vi "input_channel_to_json.vi"(1 "Analog Input Channels":T1[](array[typedef])=[{"Input Type"=enum."DAQ", "Channel Name"="Vapor Mass Flow", "Physical Channel"="cDAQ1Mod2/ai5", "Sensor Type"=enum."Mass Flow Rate", "Signal Type"=enum."Current", "Terminal Configuration"=-1, "Minimum Value"=0.004, "Maximum Value"=0.02, "TC Type"=10086, "Sensor Min"=0.0, "Sensor Max"=377.9933, "Sensor Offset"=0.0, "Sensor Unit"=enum."g/s", "Output Unit"=enum."g/s", "Unit Conversion"=1.0, "Active"=TRUE}, {"Input Type"=enum."DAQ", "Channel Name"="Vapor Line Density", "Physical Channel"="cDAQ1Mod2/ai6", "Sensor Type"=enum."Density", "Signal Type"=enum."Current", "Terminal Configuration"=-1, "Minimum Value"=0.004, "Maximum Value"=0.02, "TC Type"=10086, "Sensor Min"=0.0, "Sensor Max"=2.0, "Sensor Offset"=0.0, "Sensor Unit"=enum."g/cm3", "Output Unit"=enum."g/cm3", "Unit Conversion"=1.0, "Active"=TRUE}, {"Input Type"=enum."DAQ", "Channel Name"="Liquid Mass Flow", "Physical Channel"="cDAQ1Mod2/ai3", "Sensor Type"=enum."Mass Flow Rate", "Signal Type"=enum."Current", "Terminal Configuration"=-1, "Minimum Value"=0.004, "Maximum Value"=0.02, "TC Type"=10086, "Sensor Min"=0.0, "Sensor Max"=377.9933, "Sensor Offset"=0.0, "Sensor Unit"=enum."g/s", "Output Unit"=enum."g/s", "Unit Conversion"=1.0, "Active"=TRUE}, {"Input Type"=enum."DAQ", "Channel Name"="Liquid Line Density", "Physical Channel"="cDAQ1Mod2/ai4", "Sensor Type"=enum."Density", "Signal Type"=enum."Current", "Terminal Configuration"=-1, "Minimum Value"=0.004, "Maximum Value"=0.02, "TC Type"=10086, "Sensor Min"=0.0, "Sensor Max"=2.0, "Sensor Offset"=0.0, "Sensor Unit"=enum."g/cm3", "Output Unit"=enum."g/cm3", "Unit Conversion"=1.0, "Active"=TRUE}, {"Input Type"=enum."DAQ", "Channel Name"="Vapor Inlet Pressure DEPR", "Physical Channel"="cDAQ1Mod5/ai1", "Sensor Type"=enum."Absolute Pressure", "Signal Type"=enum."Voltage", "Terminal Configuration"=10078, "Minimum Value"=0.0, "Maximum Value"=5.0, "TC Type"=10086, "Sensor Min"=0.0, "Sensor Max"=50.0, "Sensor Offset"=0.0, "Sensor Unit"=enum."psi", "Output Unit"=enum."Pa", "Unit Conversion"=6894.75729, "Active"=FALSE}, {"Input Type"=enum."DAQ", "Channel Name"="Mega Tank Pressure", "Physical Channel"="cDAQ1Mod5/ai2", "Sensor Type"=enum."Absolute Pressure", "Signal Type"=enum."Voltage", "Terminal Configuration"=10078, "Minimum Value"=0.5, "Maximum Value"=5.5, "TC Type"=10086, "Sensor Min"=0.0, "Sensor Max"=50.0, "Sensor Offset"=0.0, "Sensor Unit"=enum."psi", "Output Unit"=enum."Pa", "Unit Conversion"=6894.75729, "Active"=TRUE}, {"Input Type"=enum."DAQ", "Channel Name"="Separator Pressure", "Physical Channel"="cDAQ1Mod5/ai0", "Sensor Type"=enum."Absolute Pressure", "Signal Type"=enum."Voltage", "Terminal Configuration"=10078, "Minimum Value"=0.0, "Maximum Value"=5.0, "TC Type"=10086, "Sensor Min"=0.0, "Sensor Max"=50.0, "Sensor Offset"=0.0, "Sensor Unit"=enum."psi", "Output Unit"=enum."Pa", "Unit Conversion"=6894.75729, "Active"=TRUE}, {"Input Type"=enum."DAQ", "Channel Name"="Liquid Inlet Pressure", "Physical Channel"="cDAQ1Mod5/ai4", "Sensor Type"=enum."Absolute Pressure", "Signal Type"=enum."Voltage", "Terminal Configuration"=10078, "Minimum Value"=0.0, "Maximum Value"=5.0, "TC Type"=10086, "Sensor Min"=0.0, "Sensor Max"=50.0, "Sensor Offset"=0.0, "Sensor Unit"=enum."psi", "Output Unit"=enum."Pa", "Unit Conversion"=6894.75729, "Active"=TRUE}, {"Input Type"=enum."DAQ", "Channel Name"="Vapor Inlet Pressure ", "Physical Channel"="cDAQ1Mod5/ai3", "Sensor Type"=enum."Absolute Pressure", "Signal Type"=enum."Voltage", "Terminal Configuration"=10078, "Minimum Value"=0.0, "Maximum Value"=5.0, "TC Type"=10086, "Sensor Min"=0.0, "Sensor Max"=50.0, "Sensor Offset"=0.0, "Sensor Unit"=enum."psi", "Output Unit"=enum."Pa", "Unit Conversion"=6894.75729, "Active"=TRUE}, {"Input Type"=enum."DAQ", "Channel Name"="Vapor Inlet Temperature", "Physical Channel"="cDAQ1Mod6/ai1", "Sensor Type"=enum."Temperature", "Signal Type"=enum."Temperature", "Terminal Configuration"=-1, "Minimum Value"=0.0, "Maximum Value"=100.0, "TC Type"=10086, "Sensor Min"=0.0, "Sensor Max"=100.0, "Sensor Offset"=0.0, "Sensor Unit"=enum."C", "Output Unit"=enum."C", "Unit Conversion"=1.0, "Active"=TRUE}, {"Input Type"=enum."DAQ", "Channel Name"="Vapor Inlet Temperature DEPR", "Physical Channel"="cDAQ1Mod7/ai0", "Sensor Type"=enum."Temperature", "Signal Type"=enum."Temperature", "Terminal Configuration"=-1, "Minimum Value"=0.0, "Maximum Value"=100.0, "TC Type"=10086, "Sensor Min"=0.0, "Sensor Max"=100.0, "Sensor Offset"=0.0, "Sensor Unit"=enum."C", "Output Unit"=enum."C", "Unit Conversion"=1.0, "Active"=FALSE}, {"Input Type"=enum."DAQ", "Channel Name"="Mega Tank Temperature", "Physical Channel"="cDAQ1Mod6/ai2", "Sensor Type"=enum."Temperature", "Signal Type"=enum."Temperature", "Terminal Configuration"=-1, "Minimum Value"=0.0, "Maximum Value"=100.0, "TC Type"=10086, "Sensor Min"=0.0, "Sensor Max"=100.0, "Sensor Offset"=0.0, "Sensor Unit"=enum."C", "Output Unit"=enum."C", "Unit Conversion"=1.0, "Active"=TRUE}, {"Input Type"=enum."DAQ", "Channel Name"="Liquid Inlet Temperature", "Physical Channel"="cDAQ1Mod7/ai3", "Sensor Type"=enum."Temperature", "Signal Type"=enum."Temperature", "Terminal Configuration"=-1, "Minimum Value"=0.0, "Maximum Value"=100.0, "TC Type"=10086, "Sensor Min"=0.0, "Sensor Max"=100.0, "Sensor Offset"=0.0, "Sensor Unit"=enum."C", "Output Unit"=enum."C", "Unit Conversion"=1.0, "Active"=TRUE}, {"Input Type"=enum."DAQ", "Channel Name"="Separator Temperature", "Physical Channel"="cDAQ1Mod6/ai0", "Sensor Type"=enum."Temperature", "Signal Type"=enum."Temperature", "Terminal Configuration"=-1, "Minimum Value"=0.0, "Maximum Value"=100.0, "TC Type"=10086, "Sensor Min"=0.0, "Sensor Max"=100.0, "Sensor Offset"=0.0, "Sensor Unit"=enum."C", "Output Unit"=enum."C", "Unit Conversion"=1.0, "Active"=TRUE}, {"Input Type"=enum."DAQ", "Channel Name"="Lower Dev Section Pressure", "Physical Channel"="cDAQ1Mod5/ai6", "Sensor Type"=enum."Absolute Pressure", "Signal Type"=enum."Voltage", "Terminal Configuration"=10078, "Minimum Value"=0.0, "Maximum Value"=5.0, "TC Type"=10086, "Sensor Min"=0.0, "Sensor Max"=60.0, "Sensor Offset"=0.0, "Sensor Unit"=enum."psi", "Output Unit"=enum."Pa", "Unit Conversion"=6894.75729, "Active"=TRUE}, {"Input Type"=enum."DAQ", "Channel Name"="Upper Dev Section Temperature", "Physical Channel"="cDAQ1Mod6/ai3", "Sensor Type"=enum."Temperature", "Signal Type"=enum."Temperature", "Terminal Configuration"=-1, "Minimum Value"=0.0, "Maximum Value"=100.0, "TC Type"=10086, "Sensor Min"=0.0, "Sensor Max"=100.0, "Sensor Offset"=0.0, "Sensor Unit"=enum."C", "Output Unit"=enum."C", "Unit Conversion"=1.0, "Active"=TRUE}, {"Input Type"=enum."DAQ", "Channel Name"="Upper Dev Section Pressure", "Physical Channel"="cDAQ1Mod5/ai5", "Sensor Type"=enum."Absolute Pressure", "Signal Type"=enum."Voltage", "Terminal Configuration"=10078, "Minimum Value"=0.0, "Maximum Value"=5.0, "TC Type"=10086, "Sensor Min"=0.0, "Sensor Max"=60.0, "Sensor Offset"=0.0, "Sensor Unit"=enum."psi", "Output Unit"=enum."Pa", "Unit Conversion"=6894.75729, "Active"=TRUE}, {"Input Type"=enum."DAQ", "Channel Name"="Test Section Temperature", "Physical Channel"="cDAQ1Mod6/ai10", "Sensor Type"=enum."Temperature", "Signal Type"=enum."Temperature", "Terminal Configuration"=-1, "Minimum Value"=0.0, "Maximum Value"=100.0, "TC Type"=10086, "Sensor Min"=0.0, "Sensor Max"=100.0, "Sensor Offset"=0.0, "Sensor Unit"=enum."C", "Output Unit"=enum."C", "Unit Conversion"=1.0, "Active"=TRUE}, {"Input Type"=enum."DAQ", "Channel Name"="Test Section Pressure", "Physical Channel"="cDAQ1Mod5/ai7", "Sensor Type"=enum."Absolute Pressure", "Signal Type"=enum."Voltage", "Terminal Configuration"=10078, "Minimum Value"=0.0, "Maximum Value"=5.0, "TC Type"=10086, "Sensor Min"=0.0, "Sensor Max"=50.0, "Sensor Offset"=0.0, "Sensor Unit"=enum."psi", "Output Unit"=enum."Pa", "Unit Conversion"=6894.75729, "Active"=TRUE}, {"Input Type"=enum."DAQ", "Channel Name"="Dwyer dP DEPR", "Physical Channel"="cDAQ1Mod5/ai9", "Sensor Type"=enum."Differential Pressure", "Signal Type"=enum."Voltage", "Terminal Configuration"=10078, "Minimum Value"=0.05, "Maximum Value"=5.05, "TC Type"=10086, "Sensor Min"=0.0, "Sensor Max"=1.0, "Sensor Offset"=0.0, "Sensor Unit"=enum."psi", "Output Unit"=enum."Pa", "Unit Conversion"=6894.75729, "Active"=FALSE}, {"Input Type"=enum."DAQ", "Channel Name"="Venturi dP", "Physical Channel"="cDAQ1Mod9/ai0", "Sensor Type"=enum."Differential Pressure", "Signal Type"=enum."Current", "Terminal Configuration"=10083, "Minimum Value"=0.00403, "Maximum Value"=0.02, "TC Type"=10086, "Sensor Min"=0.0, "Sensor Max"=10.0, "Sensor Offset"=0.0, "Sensor Unit"=enum."inH2O", "Output Unit"=enum."Pa", "Unit Conversion"=248.84, "Active"=TRUE}, {"Input Type"=enum."DAQ", "Channel Name"="PGminiPressure", "Physical Channel"="cDAQ1Mod5/ai10", "Sensor Type"=enum."Absolute Pressure", "Signal Type"=enum."Voltage", "Terminal Configuration"=10078, "Minimum Value"=0.0, "Maximum Value"=5.0, "TC Type"=10086, "Sensor Min"=0.0, "Sensor Max"=50.0, "Sensor Offset"=0.0, "Sensor Unit"=enum."psi", "Output Unit"=enum."Pa", "Unit Conversion"=6894.75729, "Active"=TRUE}, {"Input Type"=enum."DAQ", "Channel Name"="PGminiTemperature", "Physical Channel"="cDAQ1Mod7/ai6", "Sensor Type"=enum."Temperature", "Signal Type"=enum."Temperature", "Terminal Configuration"=-1, "Minimum Value"=0.0, "Maximum Value"=100.0, "TC Type"=10073, "Sensor Min"=0.0, "Sensor Max"=100.0, "Sensor Offset"=0.0, "Sensor Unit"=enum."C", "Output Unit"=enum."C", "Unit Conversion"=1.0, "Active"=TRUE}, {"Input Type"=enum."DAQ", "Channel Name"="Atmospheric Pressure", "Physical Channel"="cDAQ1Mod5/ai8", "Sensor Type"=enum."Absolute Pressure", "Signal Type"=enum."Voltage", "Terminal Configuration"=10078, "Minimum Value"=1.0, "Maximum Value"=5.0, "TC Type"=10086, "Sensor Min"=0.0, "Sensor Max"=25.0, "Sensor Offset"=0.0, "Sensor Unit"=enum."psi", "Output Unit"=enum."Pa", "Unit Conversion"=6894.75729, "Active"=TRUE}, {"Input Type"=enum."DAQ", "Channel Name"="PG Absolute Pressure", "Physical Channel"="cDAQ1Mod5/ai11", "Sensor Type"=enum."Absolute Pressure", "Signal Type"=enum."Voltage", "Terminal Configuration"=10078, "Minimum Value"=0.0, "Maximum Value"=5.0, "TC Type"=10086, "Sensor Min"=0.0, "Sensor Max"=60.0, "Sensor Offset"=0.0, "Sensor Unit"=enum."psi", "Output Unit"=enum."Pa", "Unit Conversion"=6894.75729, "Active"=TRUE}, {"Input Type"=enum."DAQ", "Channel Name"="Dwyer dP", "Physical Channel"="cDAQ1Mod2/ai7", "Sensor Type"=enum."Differential Pressure", "Signal Type"=enum."Current", "Terminal Configuration"=-1, "Minimum Value"=0.004, "Maximum Value"=0.02, "TC Type"=10086, "Sensor Min"=0.0, "Sensor Max"=500.0, "Sensor Offset"=0.0, "Sensor Unit"=enum."Pa", "Output Unit"=enum."Pa", "Unit Conversion"=1.0, "Active"=TRUE}, {"Input Type"=enum."DAQ", "Channel Name"="Mixing Tee dP DEPR", "Physical Channel"="", "Sensor Type"=enum."Differential Pressure", "Signal Type"=enum."Current", "Terminal Configuration"=-1, "Minimum Value"=0.004, "Maximum Value"=0.02, "TC Type"=10086, "Sensor Min"=0.0, "Sensor Max"=50.0, "Sensor Offset"=0.0, "Sensor Unit"=enum."psi", "Output Unit"=enum."Pa", "Unit Conversion"=6894.75729, "Active"=FALSE}, {"Input Type"=enum."DAQ", "Channel Name"="PG Vapor Temperature", "Physical Channel"="cDAQ1Mod7/ai4", "Sensor Type"=enum."Temperature", "Signal Type"=enum."Temperature", "Terminal Configuration"=-1, "Minimum Value"=0.0, "Maximum Value"=100.0, "TC Type"=10073, "Sensor Min"=0.0, "Sensor Max"=100.0, "Sensor Offset"=0.0, "Sensor Unit"=enum."C", "Output Unit"=enum."C", "Unit Conversion"=1.0, "Active"=TRUE}, {"Input Type"=enum."DAQ", "Channel Name"="PG Liquid Temperature", "Physical Channel"="cDAQ1Mod7/ai5", "Sensor Type"=enum."Temperature", "Signal Type"=enum."Temperature", "Terminal Configuration"=-1, "Minimum Value"=0.0, "Maximum Value"=100.0, "TC Type"=10073, "Sensor Min"=0.0, "Sensor Max"=100.0, "Sensor Offset"=0.0, "Sensor Unit"=enum."C", "Output Unit"=enum."C", "Unit Conversion"=1.0, "Active"=TRUE}, {"Input Type"=enum."DAQ", "Channel Name"="Window 1 to 4 dP", "Physical Channel"="cDAQ1Mod2/ai2", "Sensor Type"=enum."Differential Pressure", "Signal Type"=enum."Current", "Terminal Configuration"=-1, "Minimum Value"=0.004, "Maximum Value"=0.02, "TC Type"=10086, "Sensor Min"=0.0, "Sensor Max"=20.0, "Sensor Offset"=0.0, "Sensor Unit"=enum."inH2O", "Output Unit"=enum."Pa", "Unit Conversion"=248.84, "Active"=TRUE}, {"Input Type"=enum."DAQ", "Channel Name"="Window 1 to 7 dP", "Physical Channel"="cDAQ1Mod2/ai1", "Sensor Type"=enum."Differential Pressure", "Signal Type"=enum."Current", "Terminal Configuration"=-1, "Minimum Value"=0.004, "Maximum Value"=0.02, "TC Type"=10086, "Sensor Min"=0.0, "Sensor Max"=20.0, "Sensor Offset"=0.0, "Sensor Unit"=enum."inH2O", "Output Unit"=enum."Pa", "Unit Conversion"=248.84, "Active"=TRUE}, {"Input Type"=enum."DAQ", "Channel Name"="Window 1 to 7 Fast dP", "Physical Channel"="cDAQ1Mod2/ai0", "Sensor Type"=enum."Differential Pressure", "Signal Type"=enum."Current", "Terminal Configuration"=-1, "Minimum Value"=0.004, "Maximum Value"=0.02, "TC Type"=10086, "Sensor Min"=0.0, "Sensor Max"=2.5, "Sensor Offset"=0.0, "Sensor Unit"=enum."psi", "Output Unit"=enum."Pa", "Unit Conversion"=6894.75729, "Active"=TRUE}, {"Input Type"=enum."DAQ", "Channel Name"="Camera Voltage", "Physical Channel"="cDAQ1Mod8/ai0", "Sensor Type"=enum."Other", "Signal Type"=enum."Voltage", "Terminal Configuration"=10106, "Minimum Value"=0.0, "Maximum Value"=10.0, "TC Type"=10086, "Sensor Min"=0.0, "Sensor Max"=50.0, "Sensor Offset"=0.0, "Sensor Unit"=enum."Volt", "Output Unit"=enum."Volt", "Unit Conversion"=1.0, "Active"=TRUE}, {"Input Type"=enum."DAQ", "Channel Name"="Tinlet", "Physical Channel"="cDAQ1Mod6/ai4", "Sensor Type"=enum."Temperature", "Signal Type"=enum."Temperature", "Terminal Configuration"=-1, "Minimum Value"=0.0, "Maximum Value"=100.0, "TC Type"=10055, "Sensor Min"=-0.432, "Sensor Max"=99.438, "Sensor Offset"=0.0, "Sensor Unit"=enum."C", "Output Unit"=enum."C", "Unit Conversion"=1.0, "Active"=TRUE}, {"Input Type"=enum."DAQ", "Channel Name"="Tsectwo", "Physical Channel"="cDAQ1Mod6/ai5", "Sensor Type"=enum."Temperature", "Signal Type"=enum."Temperature", "Terminal Configuration"=-1, "Minimum Value"=0.0, "Maximum Value"=100.0, "TC Type"=10055, "Sensor Min"=-0.3803, "Sensor Max"=99.4597, "Sensor Offset"=0.0, "Sensor Unit"=enum."C", "Output Unit"=enum."C", "Unit Conversion"=1.0, "Active"=TRUE}, {"Input Type"=enum."DAQ", "Channel Name"="TS Window 1 Absolute Pressure", "Physical Channel"="cDAQ1Mod5/ai12", "Sensor Type"=enum."Absolute Pressure", "Signal Type"=enum."Voltage", "Terminal Configuration"=10078, "Minimum Value"=0.0, "Maximum Value"=5.0, "TC Type"=10086, "Sensor Min"=0.0, "Sensor Max"=50.0, "Sensor Offset"=0.0, "Sensor Unit"=enum."psi", "Output Unit"=enum."Pa", "Unit Conversion"=6894.75729, "Active"=TRUE}, {"Input Type"=enum."DAQ", "Channel Name"="TS Window 7 Absolute Pressure", "Physical Channel"="cDAQ1Mod5/ai13", "Sensor Type"=enum."Absolute Pressure", "Signal Type"=enum."Voltage", "Terminal Configuration"=10078, "Minimum Value"=0.0, "Maximum Value"=5.0, "TC Type"=10086, "Sensor Min"=0.0, "Sensor Max"=50.0, "Sensor Offset"=0.0, "Sensor Unit"=enum."psi", "Output Unit"=enum."Pa", "Unit Conversion"=6894.75729, "Active"=TRUE}, {"Input Type"=enum."DAQ", "Channel Name"="Liquid Main Diode", "Physical Channel"="cDAQ1Mod10/ai0", "Sensor Type"=enum."Other", "Signal Type"=enum."Voltage", "Terminal Configuration"=10106, "Minimum Value"=0.0, "Maximum Value"=10.0, "TC Type"=10086, "Sensor Min"=0.0, "Sensor Max"=10.0, "Sensor Offset"=0.0, "Sensor Unit"=enum."Volt", "Output Unit"=enum."Volt", "Unit Conversion"=1.0, "Active"=TRUE}, {"Input Type"=enum."DAQ", "Channel Name"="Liquid Control Diode", "Physical Channel"="cDAQ1Mod10/ai1", "Sensor Type"=enum."Other", "Signal Type"=enum."Voltage", "Terminal Configuration"=10106, "Minimum Value"=0.0, "Maximum Value"=10.0, "TC Type"=10086, "Sensor Min"=0.0, "Sensor Max"=10.0, "Sensor Offset"=0.0, "Sensor Unit"=enum."Volt", "Output Unit"=enum."Volt", "Unit Conversion"=1.0, "Active"=TRUE}, {"Input Type"=enum."DAQ", "Channel Name"="Vapor Main Diode", "Physical Channel"="cDAQ1Mod10/ai2", "Sensor Type"=enum."Other", "Signal Type"=enum."Voltage", "Terminal Configuration"=10106, "Minimum Value"=0.0, "Maximum Value"=10.0, "TC Type"=10086, "Sensor Min"=0.0, "Sensor Max"=10.0, "Sensor Offset"=0.0, "Sensor Unit"=enum."Volt", "Output Unit"=enum."Volt", "Unit Conversion"=1.0, "Active"=TRUE}, {"Input Type"=enum."DAQ", "Channel Name"="Vapor Control Diode", "Physical Channel"="cDAQ1Mod10/ai3", "Sensor Type"=enum."Other", "Signal Type"=enum."Voltage", "Terminal Configuration"=10106, "Minimum Value"=0.0, "Maximum Value"=10.0, "TC Type"=10086, "Sensor Min"=0.0, "Sensor Max"=10.0, "Sensor Offset"=0.0, "Sensor Unit"=enum."Volt", "Output Unit"=enum."Volt", "Unit Conversion"=1.0, "Active"=TRUE}, {"Input Type"=enum."DAQ", "Channel Name"="TS Exterior Temperature", "Physical Channel"="cDAQ1Mod6/ai6", "Sensor Type"=enum."Temperature", "Signal Type"=enum."Temperature", "Terminal Configuration"=-1, "Minimum Value"=0.0, "Maximum Value"=100.0, "TC Type"=10073, "Sensor Min"=-0.2775, "Sensor Max"=100.1225, "Sensor Offset"=0.0, "Sensor Unit"=enum."C", "Output Unit"=enum."C", "Unit Conversion"=1.0, "Active"=TRUE}, {"Input Type"=enum."DAQ", "Channel Name"="PG Supply Temperature", "Physical Channel"="cDAQ1Mod6/ai7", "Sensor Type"=enum."Temperature", "Signal Type"=enum."Temperature", "Terminal Configuration"=-1, "Minimum Value"=0.0, "Maximum Value"=100.0, "TC Type"=10073, "Sensor Min"=0.0, "Sensor Max"=100.0, "Sensor Offset"=0.0, "Sensor Unit"=enum."C", "Output Unit"=enum."C", "Unit Conversion"=1.0, "Active"=TRUE}, {"Input Type"=enum."DAQ", "Channel Name"="Post Mixing Tee Temperature", "Physical Channel"="cDAQ1Mod7/ai2", "Sensor Type"=enum."Temperature", "Signal Type"=enum."Temperature", "Terminal Configuration"=-1, "Minimum Value"=0.0, "Maximum Value"=100.0, "TC Type"=10073, "Sensor Min"=0.0, "Sensor Max"=1000.0, "Sensor Offset"=0.0, "Sensor Unit"=enum."Volt", "Output Unit"=enum."Volt", "Unit Conversion"=1.0, "Active"=TRUE}, {"Input Type"=enum."DAQ", "Channel Name"="Tsecthree", "Physical Channel"="cDAQ1Mod6/ai8", "Sensor Type"=enum."Temperature", "Signal Type"=enum."Temperature", "Terminal Configuration"=-1, "Minimum Value"=0.0, "Maximum Value"=100.0, "TC Type"=10055, "Sensor Min"=-0.2553, "Sensor Max"=99.6347, "Sensor Offset"=0.0, "Sensor Unit"=enum."C", "Output Unit"=enum."C", "Unit Conversion"=1.0, "Active"=TRUE}, {"Input Type"=enum."DAQ", "Channel Name"="Toutlet", "Physical Channel"="cDAQ1Mod6/ai9", "Sensor Type"=enum."Temperature", "Signal Type"=enum."Temperature", "Terminal Configuration"=-1, "Minimum Value"=0.0, "Maximum Value"=100.0, "TC Type"=10055, "Sensor Min"=-0.1957, "Sensor Max"=99.8043, "Sensor Offset"=0.0, "Sensor Unit"=enum."C", "Output Unit"=enum."C", "Unit Conversion"=1.0, "Active"=TRUE}] {"Unit Conversion" format="%0.5f"; "TC Type" items=["J"=10072, "K"=10073, "N"=10077, "R"=10082, "S"=10085, "T"=10086, "B"=10047, "E"=10055]; "Sensor Offset" format="%0.5f"; "Sensor Max" format="%0.5f"; "Sensor Min" format="%0.5f"; "Maximum Value" format="%.6f"; "Minimum Value" format="%.6f"; "Terminal Configuration" items=["Default"=-1, "RSE"=10083, "NRSE"=10078, "Differential"=10106, "Pseudodifferential"=12529]}) -> (0 "JSON string":string)   [LabVIEW 2017]
uses:
  input_channel.ctl
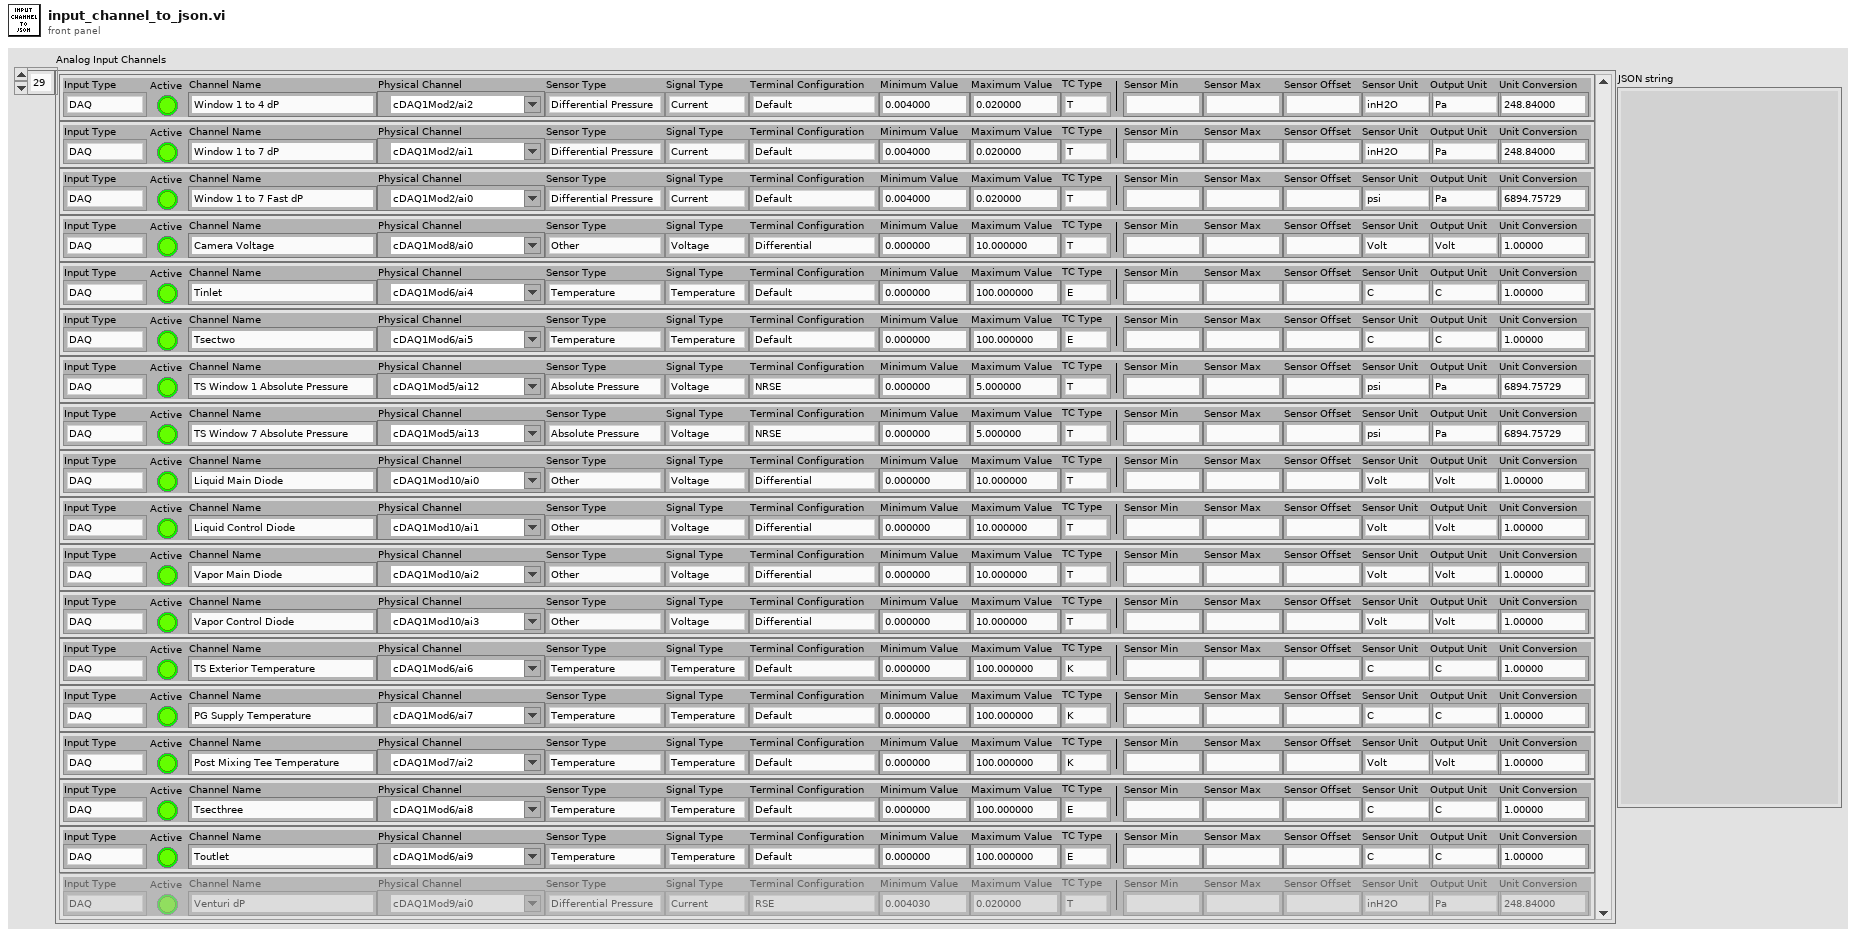
[diagram p1: front panel]
types:
  T1 = typedef "input_channel.ctl" = cluster{"Input Type":enum16{"DAQ", "Add-On"}, "Channel Name":string, "Physical Channel":tag, "Sensor Type":enum16{"Absolute Pressure", "Gauge Pressure", "Differential Pressure", "Temperature", "Mass Flow Rate", "Density", "Other"}, "Signal Type":enum16{"Voltage", "Current", "Temperature"}, "Terminal Configuration":i32, "Minimum Value":dbl, "Maximum Value":dbl, "TC Type":i32, "Sensor Min":dbl, "Sensor Max":dbl, "Sensor Offset":dbl, "Sensor Unit":enum16{"psi", "Pa", "inH2O", "inHg", "C", "K", "g/s", "g/cm3", "Volt", "Amp", ""}, "Output Unit":enum16{"psi", "Pa", "inH2O", "inHg", "C", "K", "g/s", "g/cm3", "Volt", "Amp", ""}, "Unit Conversion":dbl, "Active":bool}
  T2 = enum16{"Absolute Pressure", "Gauge Pressure", "Differential Pressure", "Temperature", "Mass Flow Rate", "Density", "Other"}
  T3 = enum16{"psi", "Pa", "inH2O", "inHg", "C", "K", "g/s", "g/cm3", "Volt", "Amp", ""}
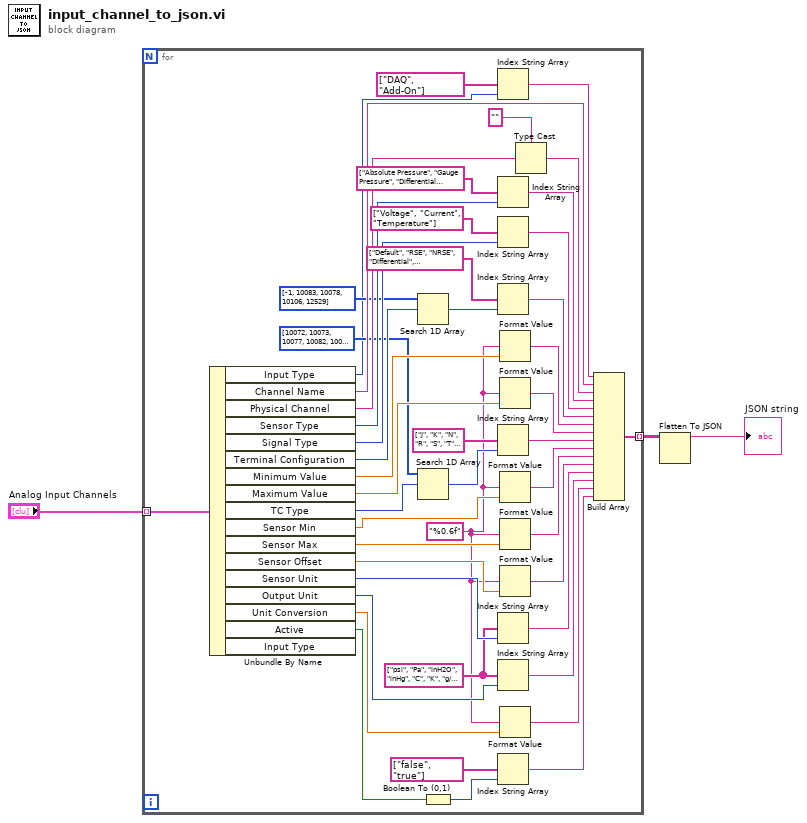
[diagram p0: block diagram]
diagram:
  n1 = for {
    tunnel: "Analog Input Channels" -> [w50] mode=indexing
    tunnel: [w7] -> w2 mode=indexing
    w18 = string[] ["psi", "Pa", "inH2O", "inHg", "C", "K", "g/s", "g/cm3", "Volt", "Amp", ""] ("Unit")
    w15 = "%0.6f" ("format string")
    n2 = Unbundle By Name(w50) -> ("Input Type"=w5:enum16{"DAQ", "Add-On"}, "Channel Name"=w48:string, "Physical Channel"=w49:tag, "Sensor Type"=w45:T2, "Signal Type"=w43:enum16{"Voltage", "Current", "Temperature"}, "Terminal Configuration"=w40:i32, "Minimum Value"=w36:dbl, "Maximum Value"=w33:dbl, "TC Type"=w30:i32, "Sensor Min"=w23:dbl, "Sensor Max"=w22:dbl, "Sensor Offset"=w21:dbl, "Sensor Unit"=w20:T3, "Output Unit"=w19:T3, "Unit Conversion"=w14:dbl, "Active"=w11:bool)  [unwired: 1 out]
    n3 = Search 1D Array(1D array=i32[] [-1, 10083, 10078, 10106, 12529] ("Array 3"), element=w40) -> (index of element=w39:i32)  [unwired: 1 in]
    n4 = Search 1D Array(1D array=i32[] [10072, 10073, 10077, 10082, 10085, 10086, 10047, 10055] ("Array 2"), element=w30) -> (index of element=w29:i32)  [unwired: 1 in]
    n5 = Boolean To (0,1)(Boolean=w11) -> (0, 1=w12:i16)
    n6 = Index String Array(1:w5, 2:string[] ["DAQ", "Add-On"] ("Input Type")) -> (0:w6:string)  [unwired: 1 in]
    n7 = Index String Array(1:w45, 2:string[] ["Absolute Pressure", "Gauge Pressure", "Differential Pressure", "Temperature", "Mass Flow Rate", "Density", "Other"] ("Sensor Type")) -> (0:w44:string)  [unwired: 1 in]
    n8 = Index String Array(1:w43, 2:string[] ["Voltage", "Current", "Temperature"] ("Signal Type")) -> (0:w41:string)  [unwired: 1 in]
    n9 = Index String Array(1:w39, 2:string[] ["Default", "RSE", "NRSE", "Differential", "Pseudodifferential"] ("Terminal Configuration")) -> (0:w35:string)  [unwired: 1 in]
    n10 = Index String Array(1:w29, 2:string[] ["J", "K", "N", "R", "S", "T", "B", "E"] ("TC Type")) -> (0:w27:string)  [unwired: 1 in]
    n11 = Index String Array(1:w20, 2:w18) -> (0:w17:string)  [unwired: 1 in]
    n12 = Index String Array(1:w19, 2:w18) -> (0:w16:string)  [unwired: 1 in]
    n13 = Index String Array(1:w12, 2:string[] ["false", "true"] ("string array")) -> (0:w9:string)  [unwired: 1 in]
    n14 = Format Value(format string=w15, value (0)=w36) -> (output string=w34:string)  [unwired: 1 in]
    n15 = Format Value(format string=w15, value (0)=w33) -> (output string=w32:string)  [unwired: 1 in]
    n16 = Format Value(format string=w15, value (0)=w23) -> (output string=w26:string)  [unwired: 1 in]
    n17 = Format Value(format string=w15, value (0)=w22) -> (output string=w25:string)  [unwired: 1 in]
    n18 = Format Value(format string=w15, value (0)=w21) -> (output string=w24:string)  [unwired: 1 in]
    n19 = Format Value(format string=w15, value (0)=w14) -> (output string=w10:string)  [unwired: 1 in]
    n20 = Type Cast(type="", x=w49) -> (*(type *) &x=w47:string)
    n21 = Build Array(w6, w48, w47, w44, w41, w35, w34, w32, w27, w26, w25, w24, w17, w16, w10, w9) -> (w7:string[])
  }
  n22 = Flatten To JSON(anything=w2) -> (JSON string=→"JSON string":string)  [unwired: 2 in, 1 out]
